vi "String to Tree Inner Part.vi"(4 "structure before":T2(array[cluster]), 5 "dummy":T1, 6 "error situation before":i32, 7 "dot or comma":string) -> (0 "error in formula-write":string, 1 "structure after":T2(array[cluster]), 2 "error situation after":i32, 3 "end of analysis":bool)   [LabVIEW 2010, in "NI_Gmath.lvlib"]
uses:
  NI_Gmath.lvlib
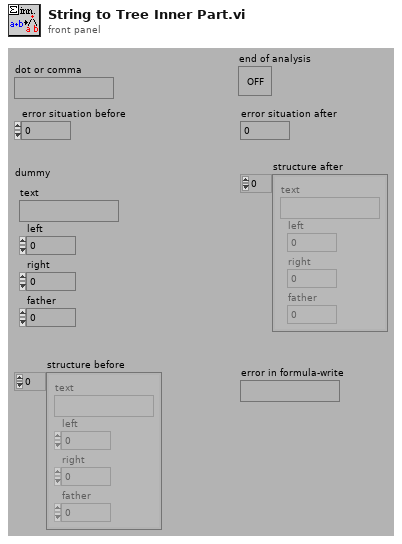
[diagram p1: front panel]
types:
  T1 = cluster{"text":string, "left":i32, "right":i32, "father":i32}
  T2 = cluster{"text":string, "left":i32, "right":i32, "father":i32}[]
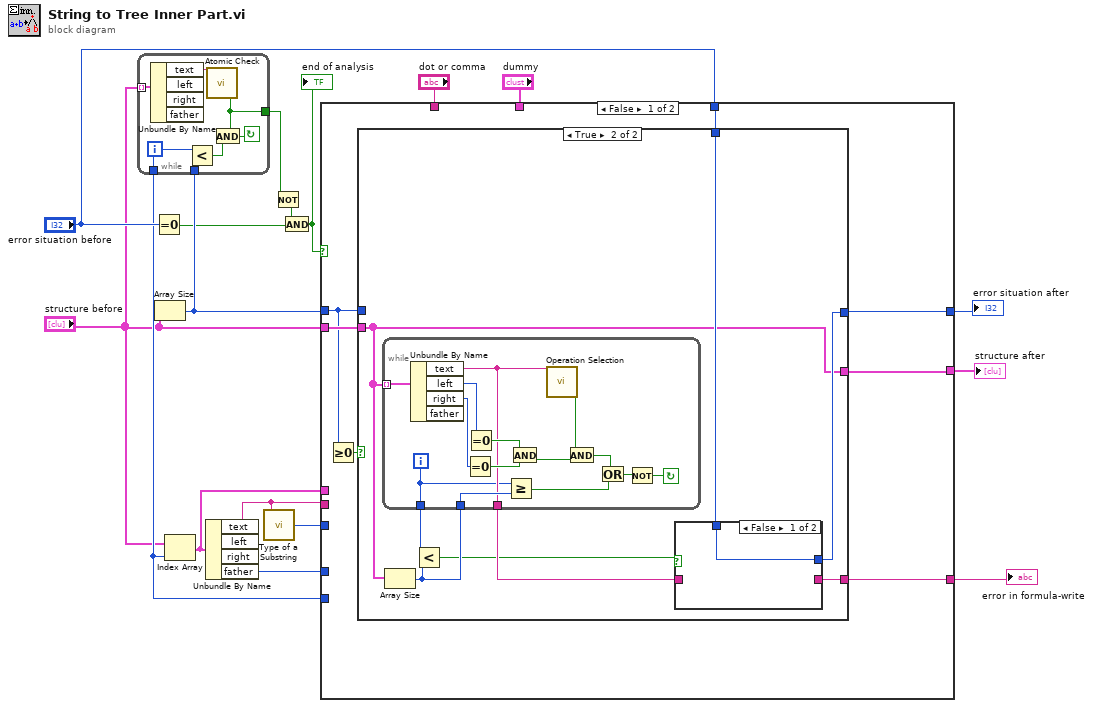
[diagram p0: block diagram]
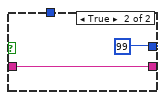
[diagram p3: hidden frame]
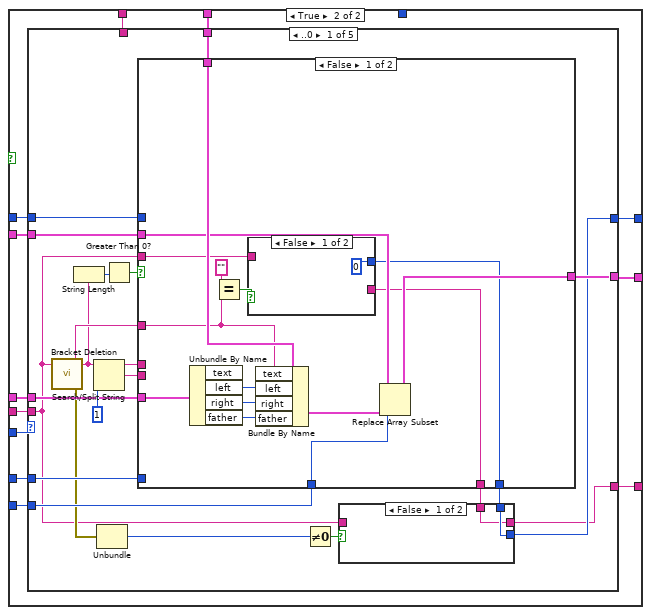
[diagram p4: hidden frame]
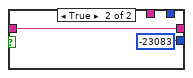
[diagram p5: hidden frame]
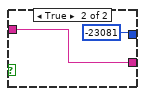
[diagram p6: hidden frame]
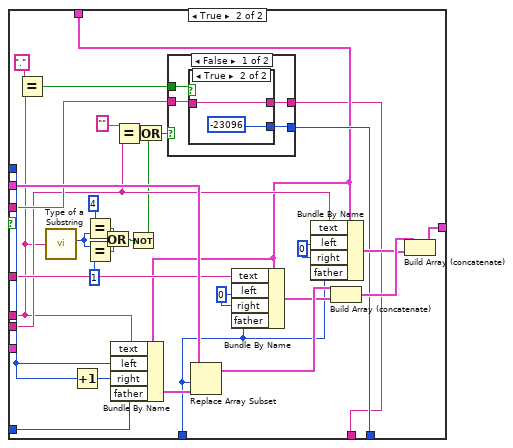
[diagram p7: hidden frame]
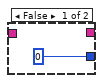
[diagram p8: hidden frame]
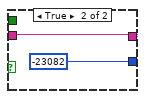
[diagram p9: hidden frame]
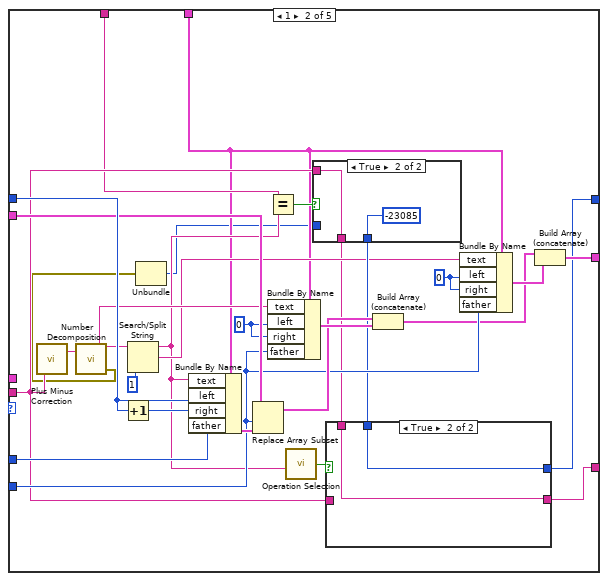
[diagram p10: hidden frame]
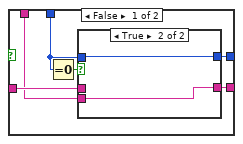
[diagram p11: hidden frame]
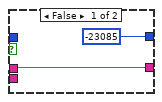
[diagram p12: hidden frame]
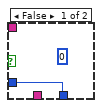
[diagram p13: hidden frame]
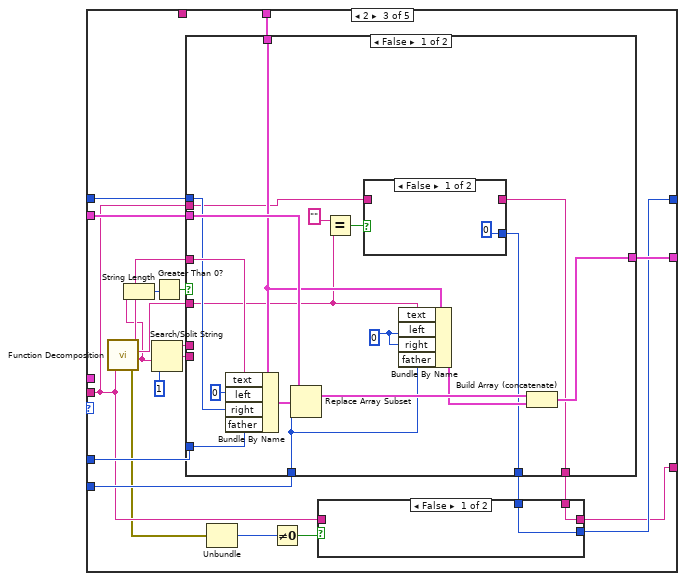
[diagram p14: hidden frame]
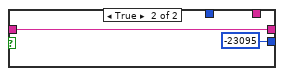
[diagram p15: hidden frame]
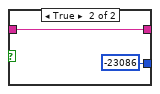
[diagram p16: hidden frame]
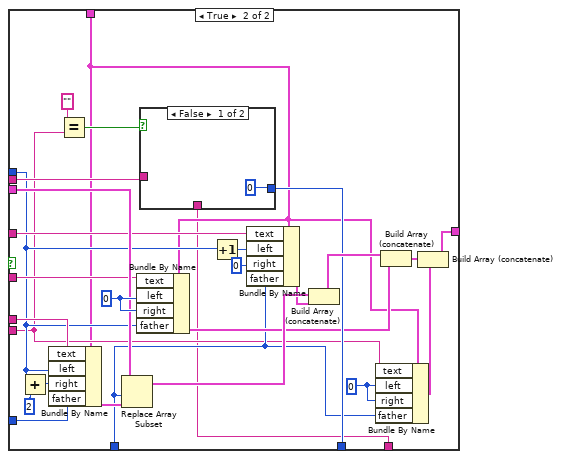
[diagram p17: hidden frame]
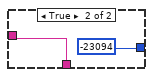
[diagram p18: hidden frame]
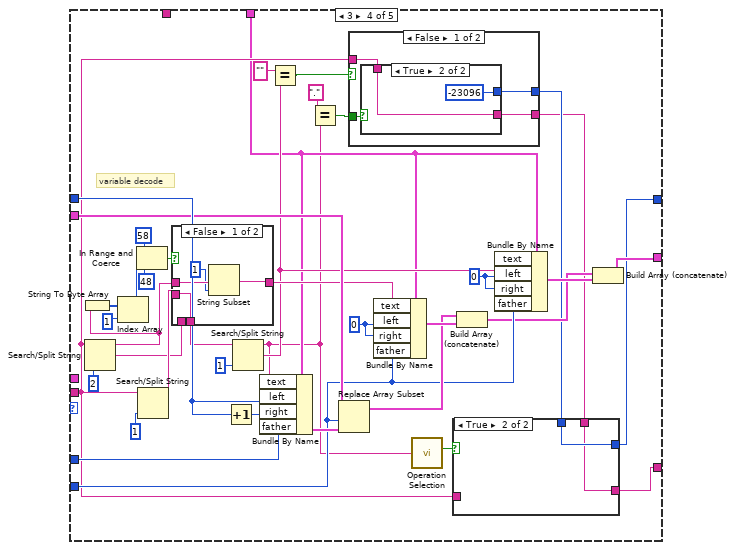
[diagram p19: hidden frame]
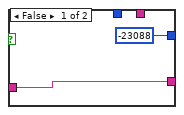
[diagram p20: hidden frame]
diagram:
  n1 = Equal To 0?(x="error situation before") -> (x = 0?=w5:bool)
  n2 = Array Size(array="structure before") -> (size(s)=w8:i32)
  n3 = while {
    tunnel: [w20] -> w9
    tunnel: w8 -> [w22]
    tunnel: [w18] -> w7
    tunnel: "structure before" -> [w24] mode=indexing
    i -> [w18]
    stop <- w19 continue-if-true
    n4 = Unbundle By Name(w24) -> ("text"=w23:string)  [unwired: 3 out]
    n5 = Less?(x=w18, y=w22) -> (x < y?=w21:bool)
    n6 = call "Atomic Check.VI"("string"=w23) -> ("atomic"=w20:bool)
    n7 = And(x=w20, y=w21) -> (x .and. y?=w19:bool)
  }
  n8 = Index Array(array="structure before", index=w7) -> (element=w10:T1)
  n9 = Unbundle By Name(w10) -> ("text"=w13:string, "father"=w6:i32)  [unwired: 2 out]
  n10 = call "Type of a Substring.VI"("item"=w13) -> ("type"=w15:i32)
  n11 = Not(x=w9) -> (.not. x?=w4:bool)
  n12 = And(x=w4, y=w5) -> (x .and. y?=w14:bool)
  "end of analysis" <- w14
  n13 = case shown="False" w14 {
    tunnel: w8 -> [w26 w70]
    tunnel: [w28 w69] -> w17
    tunnel: "structure before" -> [w31 w68]
    tunnel: w7 -> [_ w67]
    tunnel: w6 -> [_ w66]
    tunnel: w13 -> [_ w65]
    tunnel: w15 -> [_ w64]
    tunnel: w10 -> [_ w63]
    tunnel: [w30 w62] -> w11
    tunnel: "error situation before" -> [w29 _]
    tunnel: "dot or comma" -> [_ w61]
    tunnel: "dummy" -> [_ w60]
    tunnel: [w25 w59] -> w1
    frame False {
      n14 = Greater Or Equal To 0?(x=w26) -> (x >= 0?=w27:bool)
      n15 = case shown="True" w27 {
        tunnel: w29 -> [_ w39]
        tunnel: [w32 w38] -> w30
        tunnel: w31 -> [w33 w35]
        tunnel: [w33 w35] -> w28
        tunnel: w26 -> [w32 _]
        tunnel: [_ w34] -> w25
        frame False {
        }
        frame True {
          n16 = Array Size(array=w35) -> (size(s)=w41:i32)
          n17 = while {
            tunnel: w41 -> [w48]
            tunnel: [w44] -> w40
            tunnel: [w42] -> w36
            tunnel: w35 -> [w55] mode=indexing
            i -> [w42]
            stop <- w49 continue-if-true
            n18 = Unbundle By Name(w55) -> ("text"=w44:string, "left"=w54:i32, "right"=w53:i32)  [unwired: 1 out]
            n19 = Equal To 0?(x=w53) -> (x = 0?=w51:bool)
            n20 = Equal To 0?(x=w54) -> (x = 0?=w52:bool)
            n21 = Greater Or Equal?(x=w42, y=w48) -> (x >= y?=w47:bool)
            n22 = And(x=w52, y=w51) -> (x .and. y?=w50:bool)
            n23 = call "Operation Selection.VI"("selector"=w44) -> ("result"=w43:bool)
            n24 = And(x=w43, y=w50) -> (x .and. y?=w46:bool)
            n25 = Or(x=w46, y=w47) -> (x .or. y?=w45:bool)
            n26 = Not(x=w45) -> (.not. x?=w49:bool)
          }
          n27 = Less?(x=w36, y=w41) -> (x < y?=w37:bool)
          n28 = case shown="False" w37 {
            tunnel: [w56 99] -> w38
            tunnel: w39 -> [w56 _]
            tunnel: w40 -> [_ w57]
            tunnel: [_ w57] -> w34
            frame False {
            }
            frame True {
            }
          }
        }
      }
    }
    frame True {
      n29 = case shown="..0" w64 {
        tunnel: w65 -> [w76 w166 w210 w288 w338]
        tunnel: w66 -> [w91 w184 w221 w318 _]
        tunnel: w70 -> [w90 w183 w215 w317 _]
        tunnel: w67 -> [w87 w175 w219 w309 _]
        tunnel: w68 -> [w89 w180 w220 w314 w339]
        tunnel: [w85 w172 w213 w294 w339] -> w69
        tunnel: w63 -> [w80 _ _ _ _]
        tunnel: [w78 w167 w211 w289 -23087] -> w62
        tunnel: w61 -> [_ w161 _ _ _]
        tunnel: w60 -> [w73 w160 w203 w282 _]
        tunnel: [w72 w157 w202 w280 w338] -> w59
        frame ..0 {
          n30 = call "Bracket Deletion.vi"("string input with brackets"=w76) -> ("string output balanced"=w88:string, "string output rest"=w83:string, "error out"=w77:errorcluster)  [unwired: 1 in]
          n31 = String Length(string=w83) -> (length=w82:i32)
          n32 = Search/Split String(string=w83, offset (0)=1) -> (substring before match=w84:string, match + rest of string=w86:string)  [unwired: 1 in, 1 out]
          n33 = Unbundle(w77) -> ("code"=w75:i32)  [unwired: 2 out]
          n34 = Greater Than 0?(x=w82) -> (x > 0?=w81:bool)
          n35 = case shown="False" w81 {
            tunnel: w84 -> [_ w117]
            tunnel: [w103 w146] -> w85
            tunnel: w73 -> [w107 w116]
            tunnel: w86 -> [_ w130]
            tunnel: w87 -> [w104 w118]
            tunnel: w88 -> [w102 w131]
            tunnel: w89 -> [w106 w139]
            tunnel: w90 -> [_ w136]
            tunnel: w91 -> [_ w135]
            tunnel: w80 -> [w111 _]
            tunnel: w76 -> [w99 w132]
            tunnel: [w98 w133] -> w79
            tunnel: [w97 w115] -> w71
            frame False {
              n36 = Unbundle By Name(w111) -> ("left"=w110:i32, "right"=w109:i32, "father"=w108:i32)  [unwired: 1 out]
              n37 = Equal?(x="", y=w102) -> (x = y?=w100:bool)
              n38 = case shown="False" w100 {
                tunnel: w99 -> [_ w113]
                tunnel: [0 -23081] -> w98
                tunnel: [_ w113] -> w97
                frame False {
                }
                frame True {
                }
              }
              n39 = Bundle By Name(cluster=w107, "text"=w102, "left"=w110, "right"=w109, "father"=w108) -> (w105:T1)
              n40 = Replace Array Subset(array=w106, new element=w105, index=w104) -> (w103:T2)
            }
            frame True {
              w140 = 0
              w143 = 0
              n41 = Equal?(x=".", y=w117) -> (x = y?=w119:bool)
              n42 = call "Type of a Substring.VI"("item"=w117) -> ("type"=w126:i32)
              n43 = Increment(x=w136) -> (x+1=w137:i32)
              n44 = Equal?(x=4, y=w126) -> (x = y?=w125:bool)
              n45 = Equal?(x=w126, y=1) -> (x = y?=w123:bool)
              n46 = Or(x=w125, y=w123) -> (x .or. y?=w122:bool)
              n47 = Bundle By Name(cluster=w116, "text"=w117, "left"=w136, "right"=w137, "father"=w135) -> (w138:T1)
              n48 = Equal?(x="", y=w130) -> (x = y?=w124:bool)
              n49 = Not(x=w122) -> (.not. x?=w121:bool)
              n50 = Or(x=w124, y=w121) -> (x .or. y?=w128:bool)
              n51 = case shown="False" w128 {
                tunnel: [w150 -23082] -> w133
                tunnel: w132 -> [w149 w154]
                tunnel: w119 -> [w148 _]
                tunnel: [w147 w154] -> w115
                frame False {
                  n52 = case shown="True" w148 {
                    tunnel: [0 -23096] -> w150
                    tunnel: w149 -> [_ w152]
                    tunnel: [_ w152] -> w147
                    frame False {
                    }
                    frame True {
                    }
                  }
                }
                frame True {
                }
              }
              n53 = Replace Array Subset(array=w139, new element=w138, index=w118) -> (w142:T2)
              n54 = Bundle By Name(cluster=w116, "text"=w131, "left"=w140, "right"=w140, "father"=w118) -> (w141:T1)
              n55 = Bundle By Name(cluster=w116, "text"=w130, "left"=w143, "right"=w143, "father"=w118) -> (w144:T1)
              n56 = Build Array (concatenate)(w142, w141) -> (w145:T2)
              n57 = Build Array (concatenate)(w145, w144) -> (w146:T2)
            }
          }
          n58 = Not Equal To 0?(x=w75) -> (x != 0?=w74:bool)
          n59 = case shown="False" w74 {
            tunnel: [w94 -23083] -> w78
            tunnel: w76 -> [_ w95]
            tunnel: w79 -> [w94 _]
            tunnel: [w93 w95] -> w72
            tunnel: w71 -> [w93 _]
            frame False {
            }
            frame True {
            }
          }
        }
        frame 1 {
          w176 = 0
          w179 = 0
          n60 = call "Plus Minus Correction.vi"("string"=w166) -> ("new string"=w171:string)  [unwired: 1 out]
          n61 = call "Number Decomposition.VI"("number string"=w171) -> ("number"=w165:string, "rest"=w164:string, "error out"=w159:errorcluster)  [unwired: 1 in]
          n62 = Increment(x=w183) -> (x+1=w182:i32)
          n63 = Search/Split String(string=w164, offset (0)=1) -> (substring before match=w162:string, match + rest of string=w163:string)  [unwired: 1 in, 1 out]
          n64 = Unbundle(w159) -> ("code"=w158:i32)  [unwired: 2 out]
          n65 = Bundle By Name(cluster=w160, "text"=w162, "left"=w183, "right"=w182, "father"=w184) -> (w181:T1)
          n66 = Replace Array Subset(array=w180, new element=w181, index=w175) -> (w177:T2)
          n67 = Equal?(x=w161, y=w162) -> (x = y?=w170:bool)
          n68 = Bundle By Name(cluster=w160, "text"=w165, "left"=w179, "right"=w179, "father"=w175) -> (w178:T1)
          n69 = call "Operation Selection.VI"("selector"=w162) -> ("result"=w169:bool)
          n70 = case shown="True" w170 {
            tunnel: [w198 -23085] -> w168
            tunnel: w166 -> [_ w199]
            tunnel: w158 -> [w198 _]
            tunnel: [_ w199] -> w156
            frame False {
              (unwired) 0
            }
            frame True {
            }
          }
          n71 = case shown="True" w169 {
            tunnel: w168 -> [w188 w197]
            tunnel: [w190 w197] -> w167
            tunnel: w166 -> [w191 _]
            tunnel: [w187 w196] -> w157
            tunnel: w156 -> [w186 w196]
            frame False {
              n72 = Equal To 0?(x=w188) -> (x = 0?=w189:bool)
              n73 = case shown="True" w189 {
                tunnel: w191 -> [w192 _]
                tunnel: [-23085 w195] -> w190
                tunnel: w188 -> [_ w195]
                tunnel: [w192 w194] -> w187
                tunnel: w186 -> [_ w194]
                frame False {
                }
                frame True {
                }
              }
            }
            frame True {
            }
          }
          n74 = Build Array (concatenate)(w177, w178) -> (w173:T2)
          n75 = Bundle By Name(cluster=w160, "text"=w163, "left"=w176, "right"=w176, "father"=w175) -> (w174:T1)
          n76 = Build Array (concatenate)(w173, w174) -> (w172:T2)
        }
        frame 2 {
          n77 = call "Function Decomposition.VI"("function string"=w210) -> ("function text"=w216:string, "function brackets"=w214:string, "rest"=w204:string, "error out"=w207:errorcluster)  [unwired: 1 in]
          n78 = String Length(string=w204) -> (length=w209:i32)
          n79 = Search/Split String(string=w204, offset (0)=1) -> (substring before match=w218:string, match + rest of string=w217:string)  [unwired: 1 in, 1 out]
          n80 = Greater Than 0?(x=w209) -> (x > 0?=w212:bool)
          n81 = case shown="False" w212 {
            tunnel: [w235 w275] -> w213
            tunnel: w214 -> [w231 w256]
            tunnel: w203 -> [w236 w249]
            tunnel: w215 -> [w234 w253]
            tunnel: w216 -> [w243 w261]
            tunnel: w217 -> [_ w250]
            tunnel: w218 -> [_ w269]
            tunnel: w219 -> [w233 w254]
            tunnel: w220 -> [w241 w265]
            tunnel: w221 -> [w244 w263]
            tunnel: w210 -> [w229 w262]
            tunnel: [w228 w258] -> w208
            tunnel: [w227 w248] -> w201
            frame False {
              w240 = 0
              n82 = Bundle By Name(cluster=w236, "text"=w243, "left"=0, "right"=w234, "father"=w244) -> (w242:T1)
              n83 = Replace Array Subset(array=w241, new element=w242, index=w233) -> (w238:T2)
              n84 = Equal?(x="", y=w231) -> (x = y?=w230:bool)
              n85 = case shown="False" w230 {
                tunnel: w229 -> [_ w246]
                tunnel: [0 -23086] -> w228
                tunnel: [_ w246] -> w227
                frame False {
                }
                frame True {
                }
              }
              n86 = Bundle By Name(cluster=w236, "text"=w231, "left"=w240, "right"=w240, "father"=w233) -> (w237:T1)
              n87 = Build Array (concatenate)(w238, w237) -> (w235:T2)
            }
            frame True {
              w266 = 0
              w272 = 0
              n88 = Add(x=w253, y=2) -> (x+y=w251:i32)
              n89 = Bundle By Name(cluster=w249, "text"=w269, "left"=w253, "right"=w251, "father"=w263) -> (w264:T1)
              n90 = Equal?(x="", y=w250) -> (x = y?=w260:bool)
              n91 = Replace Array Subset(array=w265, new element=w264, index=w254) -> (w267:T2)
              n92 = Bundle By Name(cluster=w249, "text"=w256, "left"=w266, "right"=w266, "father"=w253) -> (w255:T1)
              n93 = case shown="False" w260 {
                tunnel: w262 -> [_ w277]
                tunnel: [0 -23094] -> w258
                tunnel: [_ w277] -> w248
                frame False {
                }
                frame True {
                }
              }
              n94 = Increment(x=w253) -> (x+1=w271:i32)
              n95 = Bundle By Name(cluster=w249, "text"=w261, "left"=w271, "right"=0, "father"=w254) -> (w257:T1)
              n96 = Build Array (concatenate)(w267, w257) -> (w268:T2)
              n97 = Bundle By Name(cluster=w249, "text"=w250, "left"=w272, "right"=w272, "father"=w254) -> (w274:T1)
              n98 = Build Array (concatenate)(w268, w255) -> (w273:T2)
              n99 = Build Array (concatenate)(w273, w274) -> (w275:T2)
            }
          }
          n100 = Unbundle(w207) -> ("code"=w206:i32)  [unwired: 2 out]
          n101 = Not Equal To 0?(x=w206) -> (x != 0?=w205:bool)
          n102 = case shown="False" w205 {
            tunnel: [w224 -23095] -> w211
            tunnel: w210 -> [_ w225]
            tunnel: w208 -> [w224 _]
            tunnel: [w223 w225] -> w202
            tunnel: w201 -> [w223 _]
            frame False {
            }
            frame True {
            }
          }
        }
        frame 3 {
          w310 = 0
          w313 = 0
          # "variable decode"
          n103 = Search/Split String(string=w288, offset (0)=2) -> (substring before match=w299:string, match + rest of string=w287:string)  [unwired: 1 in, 1 out]
          n104 = String To Byte Array(string=w299) -> (unsigned byte array=w305:u8[])
          n105 = Index Array(array=w305, index=1) -> (element=w301:u8)
          n106 = In Range and Coerce(upper limit=58, x=w301, lower limit=48) -> (In Range?=w300:bool)  [unwired: 1 out]
          n107 = Search/Split String(string=w288, offset (0)=1) -> (match + rest of string=w296:string)  [unwired: 1 in, 2 out]
          n108 = case shown="False" w300 {
            tunnel: w287 -> [_ w337]
            tunnel: [w335 w337] -> w283
            tunnel: [w332 w336] -> w298
            tunnel: w299 -> [w334 w336]
            tunnel: w296 -> [w335 _]
            frame False {
              n109 = String Subset(string=w334, length (rest)=1) -> (substring=w332:string)  [unwired: 1 in]
            }
            frame True {
            }
          }
          n110 = Increment(x=w317) -> (x+1=w316:i32)
          n111 = Search/Split String(string=w283, offset (0)=1) -> (substring before match=w281:string, match + rest of string=w284:string)  [unwired: 1 in, 1 out]
          n112 = Bundle By Name(cluster=w282, "text"=w281, "left"=w317, "right"=w316, "father"=w318) -> (w315:T1)
          n113 = Equal?(x="", y=w284) -> (x = y?=w292:bool)
          n114 = Equal?(x=".", y=w281) -> (x = y?=w285:bool)
          n115 = Replace Array Subset(array=w314, new element=w315, index=w309) -> (w311:T2)
          n116 = case shown="False" w292 {
            tunnel: [w326 -23093] -> w290
            tunnel: w288 -> [w324 w330]
            tunnel: w285 -> [w325 _]
            tunnel: [w323 w330] -> w279
            frame False {
              n117 = case shown="True" w325 {
                tunnel: [0 -23096] -> w326
                tunnel: w324 -> [_ w328]
                tunnel: [_ w328] -> w323
                frame False {
                }
                frame True {
                }
              }
            }
            frame True {
            }
          }
          n118 = Bundle By Name(cluster=w282, "text"=w298, "left"=w313, "right"=w313, "father"=w309) -> (w312:T1)
          n119 = call "Operation Selection.VI"("selector"=w281) -> ("result"=w291:bool)
          n120 = case shown="True" w291 {
            tunnel: w290 -> [_ w322]
            tunnel: [-23088 w322] -> w289
            tunnel: w288 -> [w319 _]
            tunnel: [w319 w321] -> w280
            tunnel: w279 -> [_ w321]
            frame False {
            }
            frame True {
            }
          }
          n121 = Build Array (concatenate)(w311, w312) -> (w307:T2)
          n122 = Bundle By Name(cluster=w282, "text"=w284, "left"=w310, "right"=w310, "father"=w309) -> (w308:T1)
          n123 = Build Array (concatenate)(w307, w308) -> (w294:T2)
        }
        frame 4.. {
        }
      }
    }
  }
  "structure after" <- w17
  "error situation after" <- w11
  "error in formula-write" <- w1
